vi "Read Entry Console.vi"(8 "error in (no error)":errorcluster, 11 "Car Wash Controller in":refnum<class "Car Wash Controller.lvclass">) -> (0 "error out":errorcluster, 2 "Architecture.lvlib:Queue.lvclass":refnum<class "Queue.lvclass">, 3 "Car Wash Controller out":refnum<class "Car Wash Controller.lvclass">)   [LabVIEW 2019, in "Car Wash Controller.lvlib" / "Car Wash Controller.lvclass"]
uses:
  Car Wash Controller.lvclass
  Queue/Queue.lvclass
  Car Wash Controller.lvclass/Car Wash Controller.ctl
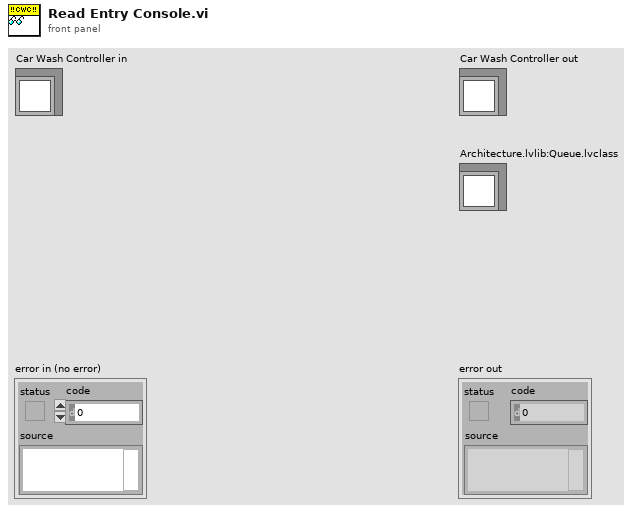
[diagram p1: front panel]
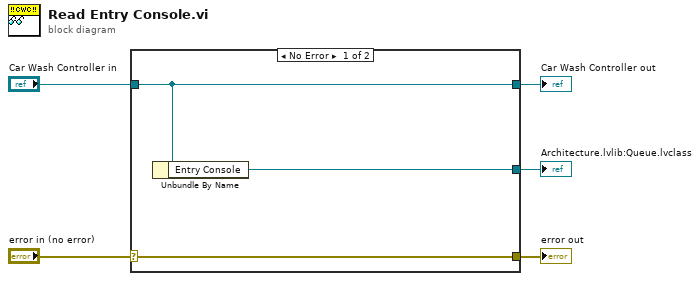
[diagram p0: block diagram]
diagram:
  n1 = case shown="No Error" "error in (no error)" {
    selector: "error in (no error)" -> [w8 w9]
    tunnel: [w8 w9] -> w4
    tunnel: [w7 w10] -> w2
    tunnel: "Car Wash Controller in" -> [w7 w10]
    tunnel: [w6 _] -> w1
    frame No Error {
      n2 = Unbundle By Name(w7) -> ("Entry Console"=w6:refnum<class "Queue.lvclass">)
    }
    frame Error {
    }
  }
  "error out" <- w4
  "Car Wash Controller out" <- w2
  "Architecture.lvlib:Queue.lvclass" <- w1
